vi "Planta.vi"(0 "u":dbl=0.1, 1 "R":dbl=0.0295 min=0.0 max=100.0 step=1.0, 2 "r":dbl=0.0015, 3 "dt":dbl=0.05 format="%0.2f") -> (5 "h":dbl format="%0.2f")   [LabVIEW 2010]
uses:
  <vilib>/ptbypt/NI_PtbyPt.lvlib
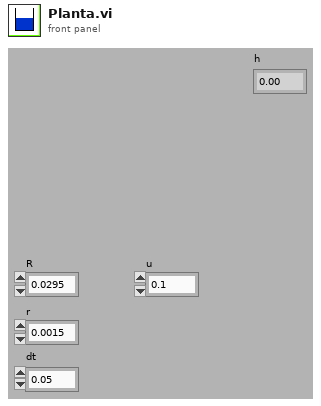
[diagram p1: front panel]
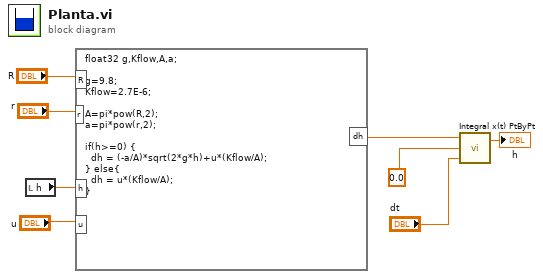
[diagram p0: block diagram]
diagram:
  n1 = local read "h"() -> (w1:dbl)
  n2 = formula code="float32 g,Kflow,A,a;\n\ng=9.8;\nKflow=2.7E-6;\n\nA=pi*pow(R,2);\na=pi*pow(r,2);\n\nif(h>=0) {\n  dh = (-a/A)*sqrt(2*g*h)+u*(Kflow/A);\n} else{ \n  dh = u*(Kflow/A);\n}"("R"="R", "r"="r", "h"=w1, "u"="u") -> ("dh"=w6:dbl)
  n3 = call <vilib>:"Integral x(t) PtByPt.vi"("dt"="dt", "initial condition"=0.0, "x"=w6) -> ("integral x(t)"=→"h":dbl)  [unwired: 1 in, 1 out]
